vi "Get DDG External Output Polarity.vi"(10 "puiPolarity":u32, 11 "uiIndex":u32) -> (2 "puiPolarity out":u32, 3 "function return":u32)   [LabVIEW 2018, in "AndorSDK.lvlib"]
doc: "EXPNETTYPE unsigned int WINAPI GetDDGExternalOutputPolarity(at_u32 uiIndex, at_u32 * puiPolarity);"
uses:
  AndorSDK.lvlib
  ATMCD32D.dll
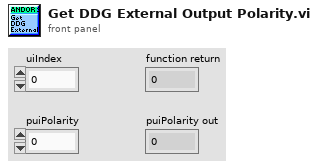
[diagram p1: front panel]
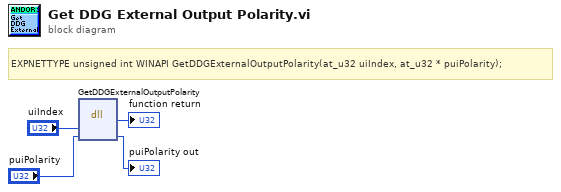
[diagram p0: block diagram]
diagram:
  # "EXPNETTYPE unsigned int WINAPI GetDDGExternalOutputPolarity(at_u32 uiIndex, at_u32 * puiPolarity);"
  n1 = dll-call lib="PTH2babs E\nPersönliches02 - Arbeit03-HiwijobsLabviewCodelibANDOR\tAndor SDK\nATMCD32D.*" fn="GetDDGExternalOutputPolarity"("uiIndex"="uiIndex", "puiPolarity"="puiPolarity") -> (→"function return":u32, "puiPolarity"=→"puiPolarity out":u32)  [unwired: 4 in, 2 out]
